vi "Configure Analog Alarm Type.vi"(7 "Unit Address (1)":u8=1, 8 "error in (no error)":errorcluster, 9 "Alarm Type (0: No Alarm)":u8(ring) items=["No Alarm", "Absolute High", "Absolute Low", "Deviation High", "Deviation Low", "Deviation Band", "Rising Rate of Change Alarm", "Falling Rate of Change Alarm"], 10 "Alarm Number (1)":u16=1 min=1 max=8, 11 "VISA resource name":refnum<visa-resource-name>) -> (0 "error out":errorcluster, 3 "VISA resource name out":refnum<visa-resource-name>)   [LabVIEW 2014, in "Eurotherm 35xx Series.lvlib"]
doc: "This VI configure analog alarm type.\nThe type of alarm determines when it will be triggered. Examples are a full scale high, where the input value has to be higher than the threshold to set the alarm off.\n\nWarning: This VI uses Controller Configuration Mode, this interrupts working process (device will not control).\nIt is recommended that the device should be disconnected from any active process."
uses:
  <instrlib>/Eurotherm 35xx Series/Eurotherm 35xx Series.lvlib
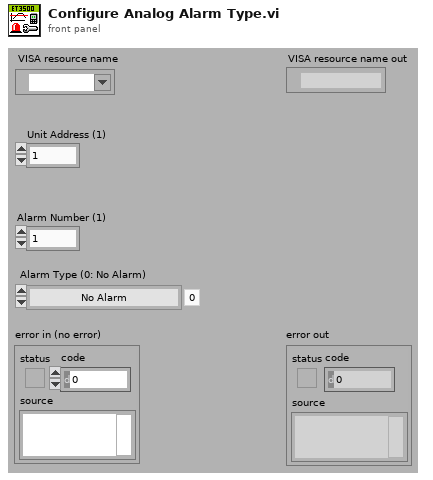
[diagram p1: front panel]
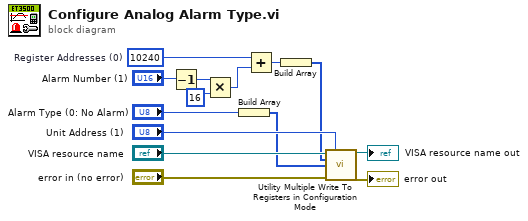
[diagram p0: block diagram]
diagram:
  w10 = 10240  # Register Addresses (0)
  n1 = Decrement(x="Alarm Number (1)") -> (x-1=w13:u16)
  n2 = Multiply(x=w13, y=u16 16) -> (x*y=w11:u16)
  n3 = Build Array("Alarm Type (0: No Alarm)") -> (w3:u8[])
  n4 = Add(x=w10, y=w11) -> (x+y=w2:i32)
  n5 = Build Array(w2) -> (w1:i32[])
  n6 = call <instrlib>:"Utility Multiple Write To Registers in Configuration Mode.vi"("VISA resource name"="VISA resource name", "Unit Address (1)"="Unit Address (1)", "Registers Addresses (0)"=w1, "Data (0)"=w3, "error in (no error)"="error in (no error)") -> ("VISA resource name out"=→"VISA resource name out":refnum<visa-resource-name>, "error out"=→"error out":errorcluster)  [unwired: 9 in]
